vi "Save_Data.vi"(8 "error in (no error)":errorcluster, 11 "Analysis in":refnum<class "Analysis.lvclass">) -> (0 "error out":errorcluster, 3 "Analysis out":refnum<class "Analysis.lvclass">)   [LabVIEW 2015]
doc: "Saves the data stored in the AnalysisObject according to the type of DataSource either in a file or in a DB.\n\nFor Text Files:\nThe Content of the original file is comletely rewritten, using the same function that saves the data in MSControl."
uses:
  MSControl/Classes/Analysis/Analysis.lvclass
  global_variables.vi
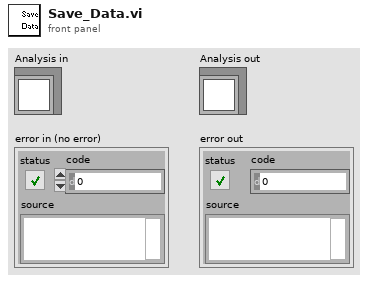
[diagram p1: front panel]
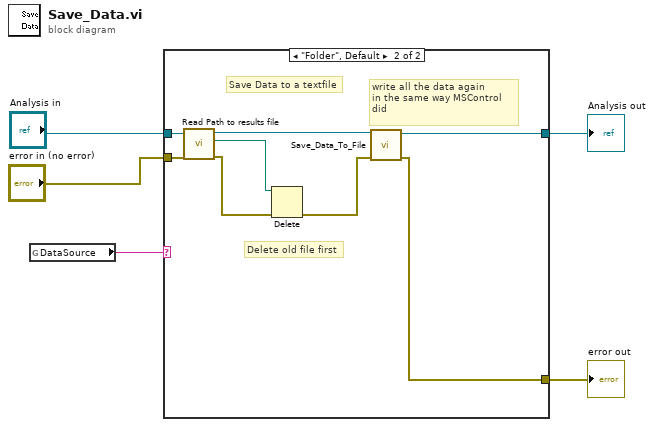
[diagram p0: block diagram]
diagram:
  n1 = global read "global_variables.vi" "DataSource"() -> (w1:string)
  n2 = case shown="\"Folder\", Default" w1 {
    tunnel: [w6 w14] -> w5
    tunnel: [w7 w15] -> w4
    tunnel: "error in (no error)" -> [w6 w12]
    tunnel: "Analysis in" -> [w7 w13]
    frame "Database" {
      # "SAve Data to a database record"
    }
    frame "Folder", Default {
      # "write all the data again\nin the same way MSControl\ndid"
      # "Delete old file first"
      # "Save Data to a textfile"
      n3 = call-dynamic "Read Path to results file.vi"("error in (no error)"=w12, "Analysis in"=w13) -> ("error out"=w10:errorcluster, "Path to results file"=w9:path, "Analysis out"=w11:refnum<class "Analysis.lvclass">)  [unwired: 7 in]
      n4 = Delete(path (use dialog)=w9, error in=w10) -> (error out=w8:errorcluster)  [unwired: 3 in, 2 out]
      n5 = call "Save_Data_To_File.vi"("error in (no error)"=w8, "Analysis in"=w11) -> ("error out"=w14:errorcluster, "Analysis out"=w15:refnum<class "Analysis.lvclass">)  [unwired: 8 in]
    }
  }
  "error out" <- w5
  "Analysis out" <- w4
